vi "I2C Master.vi"(2 "error in (no error)":errorcluster, 3 "Arduino Mode":T1=enum."Mode 0") -> (0 "I2C Error":errorcluster, 1 "Arduino Data":T2)   [LabVIEW 2018]
uses:
  I2C MASTER Type Def.ctl
  <vilib>/Studica/Studica Toolkit/Background/I2C Channel.ctl
panel:
  out "Compass High Byte":u8
  out "Compass Low Byte":u8
  out "Right Ultrasonic":u8
  out "Left Ultrasonic":u8
  out "Arduino Status":u8
  out "Front Left Ultrasonic":u8
  out "Front Right Ultrasonic":u8
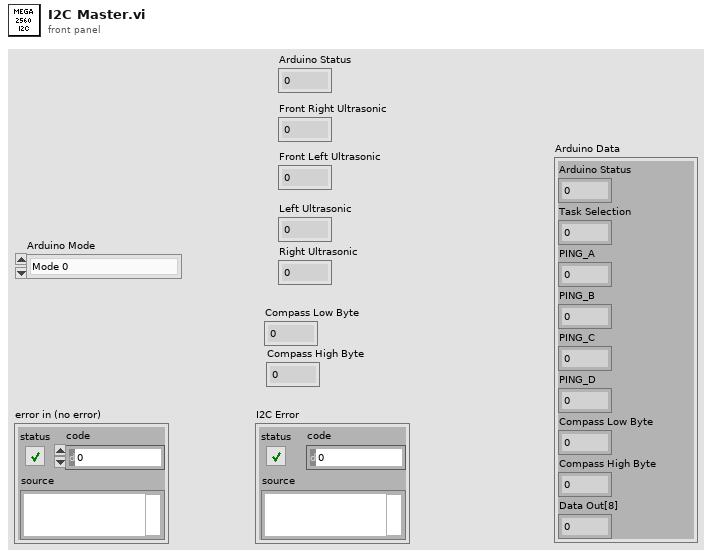
[diagram p1: front panel]
types:
  T1 = typedef "I2C MASTER Type Def.ctl" = enum16{"Last State", "Mode 0", "Mode 1", "Mode 2", "Mode 3", "Mode 4", "Mode 5", "Mode 6", "Mode 7", "Mode 8", "Mode 9", "Mode 10"}
  T2 = cluster{"Arduino Status":u8, "Task Selection":u8, "PING_A":u8, "PING_B":u8, "PING_C":u8, "PING_D":u8, "Compass Low Byte":u8, "Compass High Byte":u8, "Data Out[8]":u8}
  T3 = typedef "I2C Channel.ctl" = enum16{"Not Connected", "A", "B"}
  T4 = cluster{"I2C Channel":T3, "FPGA VI Reference Out":refnum<k20>}
  T5 = cluster{"Data Out[0]":u8, "Data Out[1]":u8, "Data Out[2]":u8, "Data Out[3]":u8, "Data Out[4]":u8, "Data Out[5]":u8, "Data Out[6]":u8, "Data Out[7]":u8, "Data Out[8]":u8}
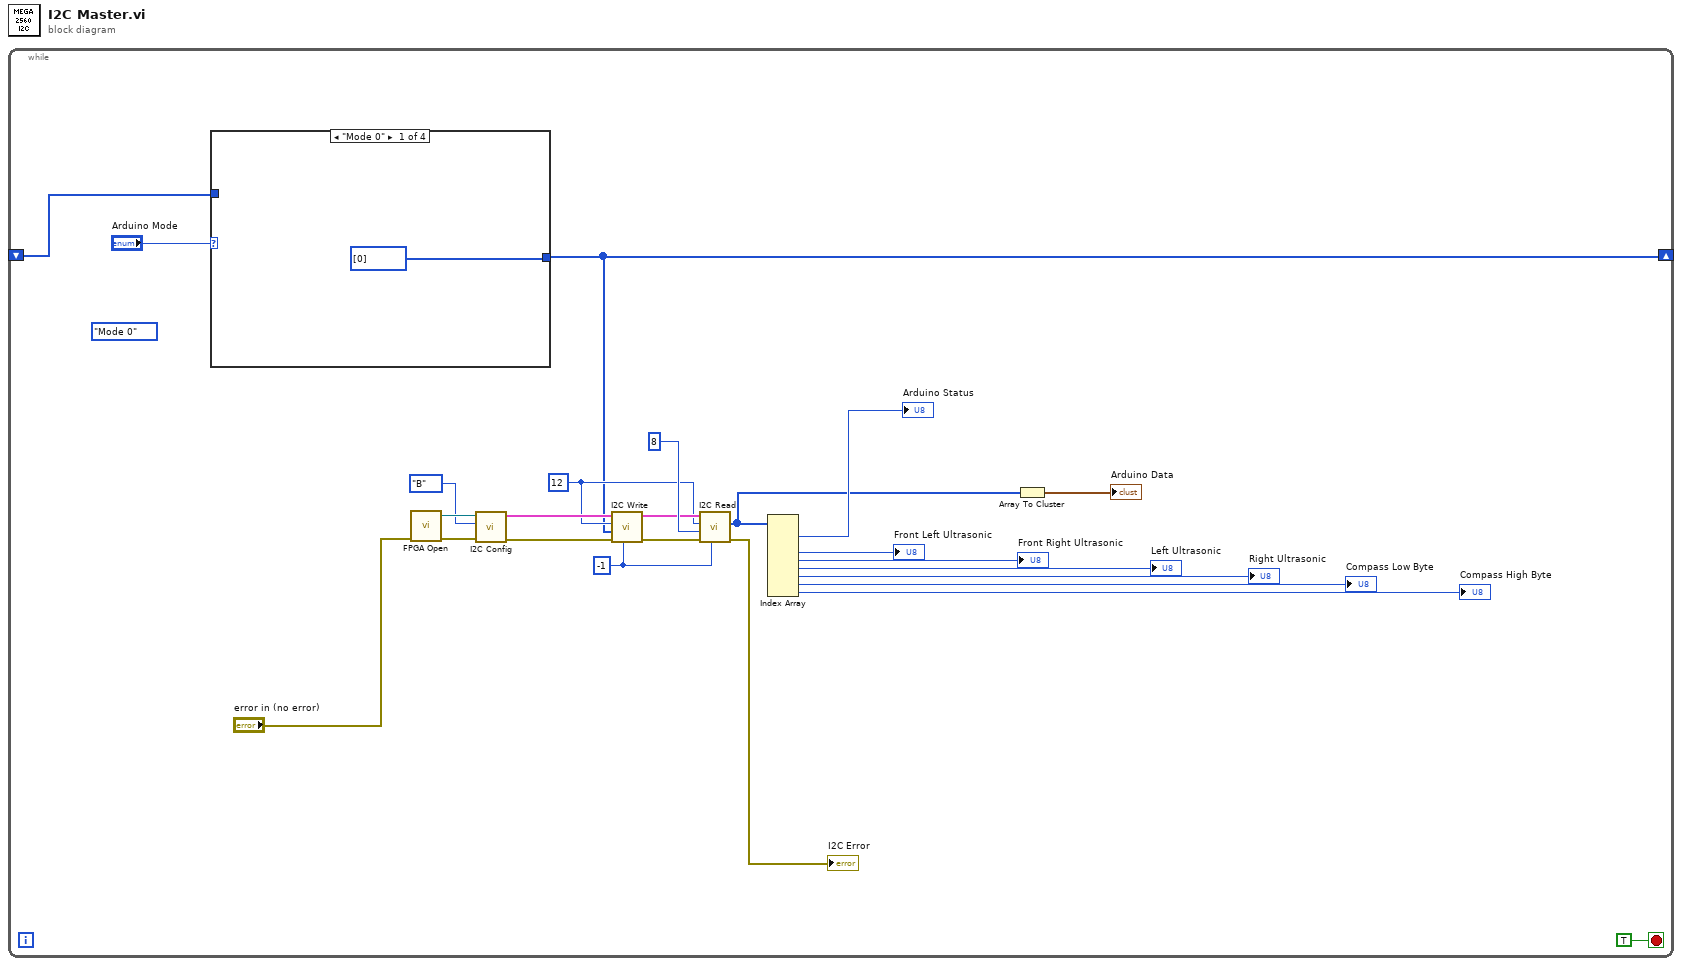
[diagram p0: block diagram]
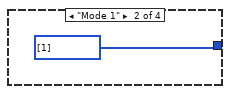
[diagram p2: hidden frame]
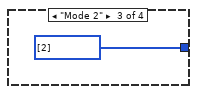
[diagram p3: hidden frame]
diagram:
  n1 = while {
    shift-right: [w3] -> _
    shift-left: _ -> [w1]
    stop <- TRUE stop-if-true
    (unwired) I2C_MASTER_Type_Def."Mode 0" ("Arduino Mode")
    w16 = -1 ("Timeout ms (1000)")
    w17 = u8 12 ("Slave Address (7-bit)")
    n2 = case shown="\"Mode 0\"" "Arduino Mode" {
      tunnel: [u8[] [0] ("Data to Write") u8[] [1] ("Data to Write") u8[] [2] ("Data to Write") w29] -> w3
      tunnel: w1 -> [_ _ _ w29]
      frame "Mode 0" {
      }
      frame "Mode 1" {
      }
      frame "Mode 2" {
      }
      frame "Last State", Default {
      }
    }
    n3 = call <vilib>:"FPGA Open.vi"("error in (no error)"="error in (no error)") -> ("error out"=w23:errorcluster, "FPGA Reference Out"=w24:refnum<k20>)  [unwired: 9 in]
    n4 = call <vilib>:"I2C Config.vi"("error in (no error)"=w23, "I2C Channel"=I2C_Channel."B", "FPGA Reference"=w24) -> ("error out"=w21:errorcluster, "I2C Ref Out"=w25:T4)  [unwired: 7 in]
    n5 = call <vilib>:"I2C Write.vi"("Timeout ms (1000)"=w16, "error in (no error)"=w21, "Data to Write"=w3, "Slave Address (7-bit)"=w17, "I2C Ref In"=w25) -> ("error out"=w19:errorcluster, "I2C Ref Out"=w18:T4)  [unwired: 5 in]
    n6 = call <vilib>:"I2C Read.vi"("Timeout ms (1000)"=w16, "error in (no error)"=w19, "Bytes to Read"=u32 8, "Slave Address (7-bit)"=w17, "I2C Ref In"=w18) -> ("error out"=→"I2C Error":errorcluster, "Data Out"=w10:u8[])  [unwired: 4 in, 1 out]
    n7 = Index Array(array=w10) -> (element #1=→"Arduino Status":u8, element #3=→"Front Left Ultrasonic":u8, element #4=→"Front Right Ultrasonic":u8, element #5=→"Left Ultrasonic":u8, element #6=→"Right Ultrasonic":u8, element #7=→"Compass Low Byte":u8, element #8=→"Compass High Byte":u8)  [unwired: 8 in, 1 out]
    n8 = Array To Cluster(array=w10) -> (cluster=→"Arduino Data":T5)
  }
